vi "Main.vi"(11 "Module Admin":refnum<class "Delacor_lib_QMH_Cloneable Module Admin.lvclass">) -> ()   [LabVIEW 2025, in "Motor.lvlib"]
doc: "This template is based off of the Queued Message Handler design pattern and the Queued Message Handler project template that ships with LabVIEW.\n\nThe main difference is that the queue is private to this module and communication between modules is performed via Broadcast and Request events.\n\nRequest events are wrapped in public API methods and are handled in the Event Handling Loop (EHL) of this VI. Any module can register for Broadcast events sent by this module. The EHL generates messages based on user interface actions.\n\nThe Message Handling Loop (MHL) processes messages generated by the EHL, or by other messages. The messages are string values, so new messages can be added easily to the Message Cases case structure in the MHL. Each message cluster can also provide an optional value for Message Data, which is a variant that can be converted to whatever message-specific data is required.\n_____\nBased on DQMH Dev Tools: Project Template 7.1.2.1547."
uses:
  Motor.lvlib
  <vilib>/Delacor/Delacor QMH/Libraries/Message Queue_class/Delacor_lib_QMH_Message Queue.lvclass
  Module Data--cluster.ctl
  <vilib>/Utility/miscctls.llb/LVPointTypeDef.ctl
  <vilib>/Delacor/Delacor QMH/Libraries/Message Queue_class/Delacor_lib_QMH_Enqueue Message (Single).vi
  Stop Argument--cluster.ctl
  <vilib>/Delacor/Delacor QMH/Libraries/Cloneable Module Admin_class/Delacor_lib_QMH_Cloneable Module Admin.lvclass
  close (Reply Payload)--cluster.ctl
  close Argument--cluster.ctl
  Classes/Stepper/Stepper.lvclass
  init (Reply Payload)--cluster.ctl
  init Argument--cluster.ctl
  clear error (Reply Payload)--cluster.ctl
  clear error Argument--cluster.ctl
  read config (Reply Payload)--cluster.ctl
  read config Argument--cluster.ctl
  read position (Reply Payload)--cluster.ctl
  read position Argument--cluster.ctl
  go to position (Reply Payload)--cluster.ctl
  go to position Argument--cluster.ctl
  jog motor (Reply Payload)--cluster.ctl
  jog motor Argument--cluster.ctl
  select child (Reply Payload)--cluster.ctl
  Classes/Stepper/Motor Selection.ctl
  select child Argument--cluster.ctl
  Classes/CL57RS/CL57RS.lvclass
  C:/Users/Tyson.Grover/Desktop/Repositories/torque-test-station/Libraries/Motor/Classes/Stepper/Stepper.lvclass
  C:/Users/Tyson.Grover/Desktop/Repositories/torque-test-station/Libraries/Motor/Classes/CL57RS/CL57RS.lvclass
panel:
  out "error out":errorcluster
  out "Status":string
  in  "Simulate EHL Error":bool
  in  "Simulate MHL Error":bool
  # "Other processes communicate with this Module via its Public API (wrappers for its Request Events).\n\nThis Module communicates with other processes via its Broadcast Events.\nAny process that wants to receive these messages can register for this module's Broadcast events."
  # "This template is for the DQMH framework. See the block diagram for more information on how to use this template."
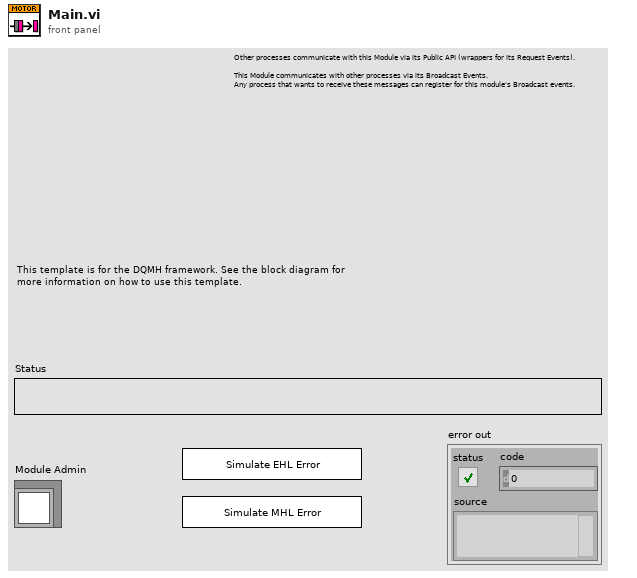
[diagram p1: front panel]
types:
  T1 = typedef "Motor.lvlib/Request Events--cluster.ctl" = cluster{"Stop Module":refnum<user-event>, "Show Panel":refnum<user-event>, "Hide Panel":refnum<user-event>, "Show Diagram":refnum<user-event>, "Get Module Execution Status":refnum<user-event>, "close":refnum<user-event>, "init":refnum<user-event>, "clear error":refnum<user-event>, "read config":refnum<user-event>, "read position":refnum<user-event>, "go to position":refnum<user-event>, "jog motor":refnum<user-event>, "select child":refnum<user-event>}
  T2 = typedef "Motor.lvlib/Module Data--cluster.ctl" = cluster{"Status":string, "Motor Object":refnum<class "Stepper.lvclass">}
  T3 = enum32{"invalid lock state", "Not Locked", "Locked (No Password)", "Password-protected"}
  T4 = typedef "Motor.lvlib/Stop Argument--cluster.ctl" = cluster{"Module ID":i32, "Origin":string, "Exit via Stop Module Req?":bool, "Wait for Module to stop?":bool}
  T5 = typedef "Motor.lvlib/close Argument--cluster.ctl" = cluster{"Module ID":i32, "Wait Notifier":refnum<notifier>, "wait for reply":bool}
  T6 = typedef "Motor.lvlib/init Argument--cluster.ctl" = cluster{"Module ID":i32, "Wait Notifier":refnum<notifier>, "wait for reply":bool}
  T7 = typedef "Motor.lvlib/clear error Argument--cluster.ctl" = cluster{"Module ID":i32, "Wait Notifier":refnum<notifier>, "wait for reply":bool}
  T8 = typedef "Motor.lvlib/read config Argument--cluster.ctl" = cluster{"Module ID":i32, "json file path":path, "Wait Notifier":refnum<notifier>, "wait for reply":bool}
  T9 = typedef "Motor.lvlib/read position Argument--cluster.ctl" = cluster{"Module ID":i32, "Wait Notifier":refnum<notifier>, "wait for reply":bool}
  T10 = typedef "Motor.lvlib/go to position Argument--cluster.ctl" = cluster{"Module ID":i32, "Position":dbl, "Velocity [rpm]":i32, "Pause Time [ms]":i32, "Wait Notifier":refnum<notifier>, "wait for reply":bool}
  T11 = typedef "Motor.lvlib/jog motor Argument--cluster.ctl" = cluster{"Module ID":i32, "CCW? (T)":bool, "Speed [rpm]":dbl, "Wait Notifier":refnum<notifier>, "wait for reply":bool}
  T12 = typedef "Motor.lvlib/select child Argument--cluster.ctl" = cluster{"Module ID":i32, "Enum":T13, "Wait Notifier":refnum<notifier>, "wait for reply":bool}
  T13 = typedef "Motor Selection.ctl" = enum16{"Stepper", "CL57RS"}
  T14 = typedef "LVPointTypeDef.ctl" = cluster{"Horizontal":i16, "Vertical":i16}
  T15 = enum32{"Invalid", "Standard", "Closed", "Hidden", "Minimized", "Maximized"}
  T16 = typedef "Motor.lvlib/close (Reply Payload)--cluster.ctl" = cluster{"Module ID":i32, "error":errorcluster}
  T17 = typedef "Motor.lvlib/init (Reply Payload)--cluster.ctl" = cluster{"Module ID":i32, "error":errorcluster}
  T18 = typedef "Motor.lvlib/clear error (Reply Payload)--cluster.ctl" = cluster{"Module ID":i32, "error":errorcluster}
  T19 = typedef "Motor.lvlib/read config (Reply Payload)--cluster.ctl" = cluster{"Module ID":i32, "error":errorcluster}
  T20 = typedef "Motor.lvlib/read position (Reply Payload)--cluster.ctl" = cluster{"Module ID":i32, "Position":dbl, "error":errorcluster}
  T21 = typedef "Motor.lvlib/go to position (Reply Payload)--cluster.ctl" = cluster{"Module ID":i32, "Position":dbl, "error":errorcluster}
  T22 = typedef "Motor.lvlib/jog motor (Reply Payload)--cluster.ctl" = cluster{"Module ID":i32, "Position":dbl, "error":errorcluster}
  T23 = typedef "Motor.lvlib/select child (Reply Payload)--cluster.ctl" = cluster{"Module ID":i32, "error":errorcluster}
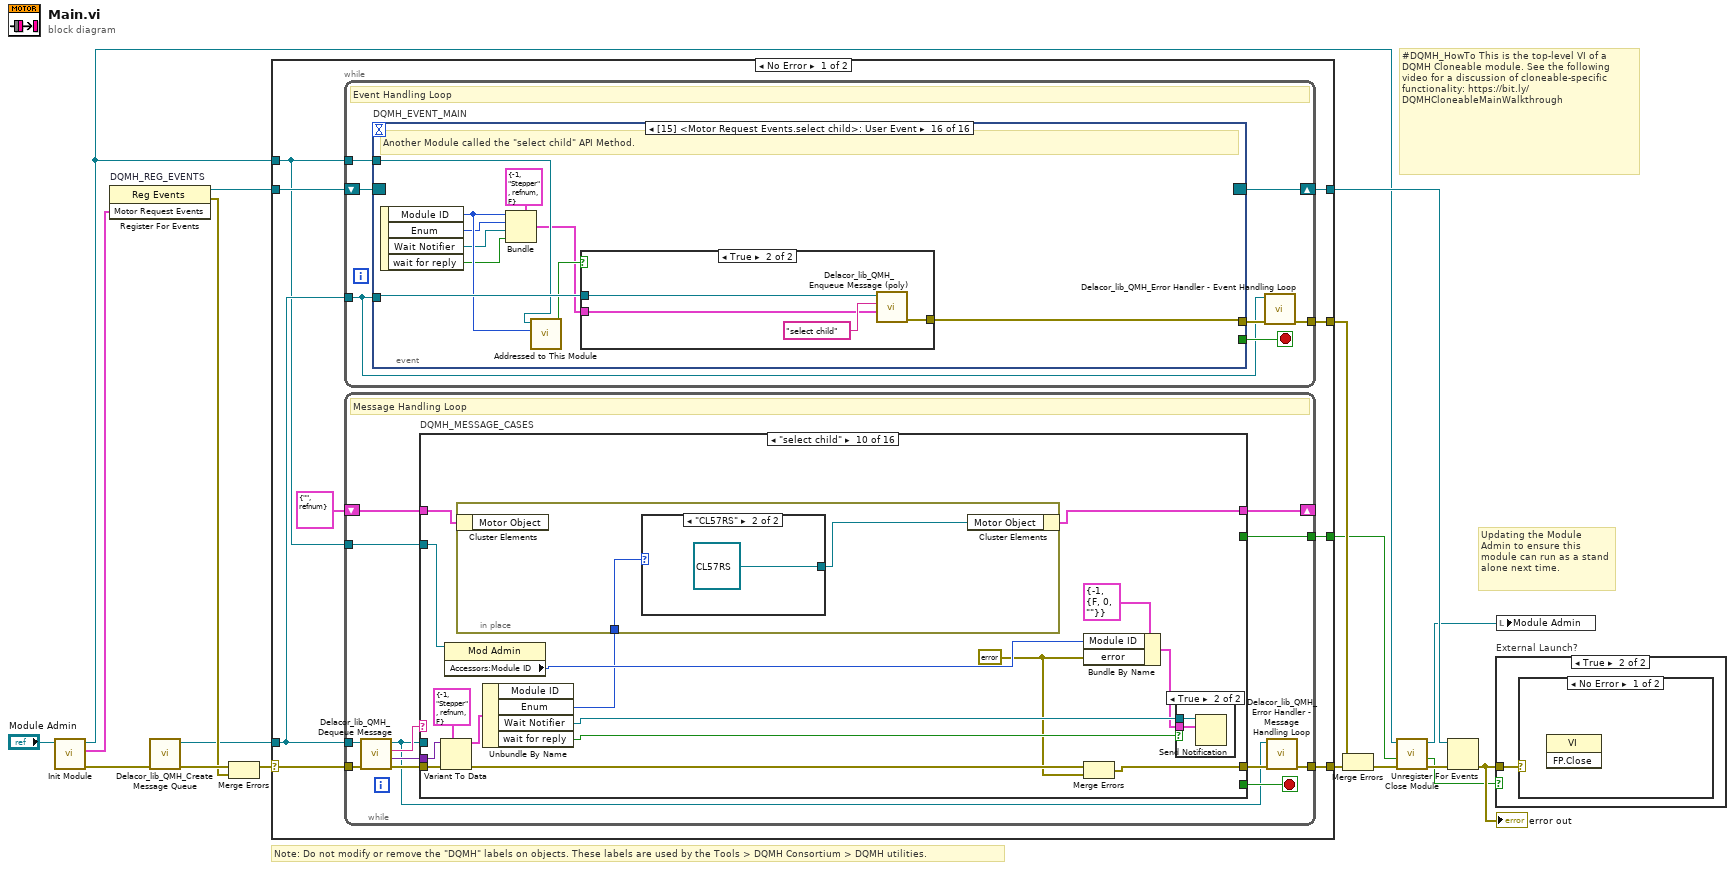
[diagram p0: block diagram]
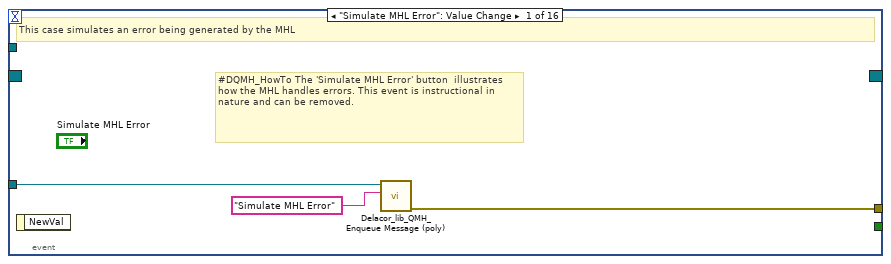
[diagram p2: hidden frame]
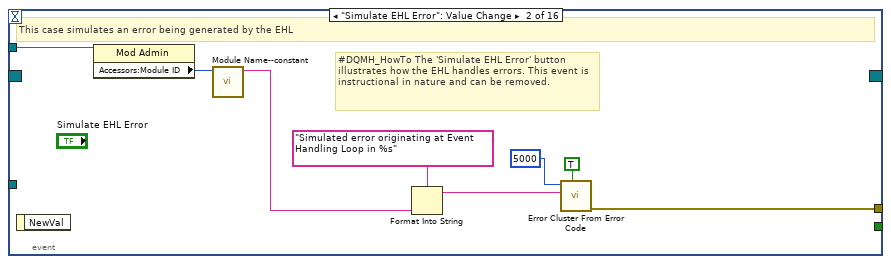
[diagram p3: hidden frame]
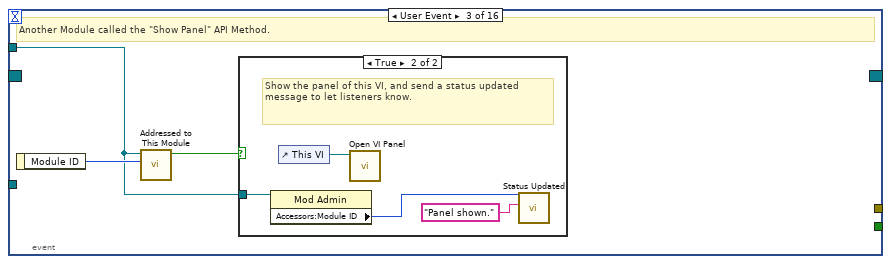
[diagram p4: hidden frame]
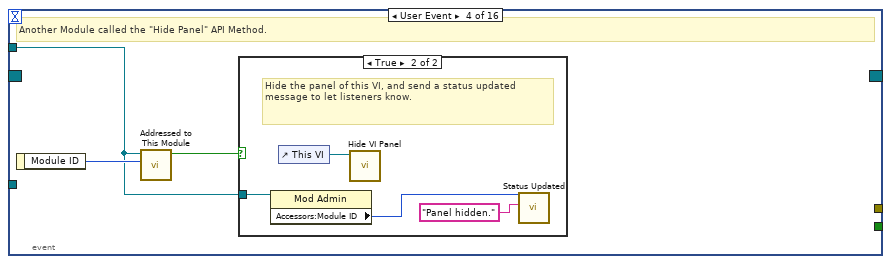
[diagram p6: hidden frame]
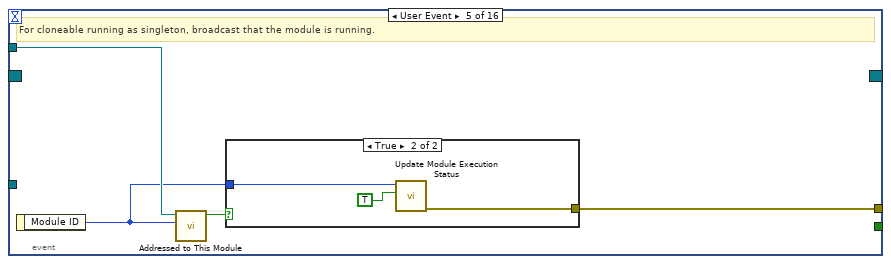
[diagram p8: hidden frame]
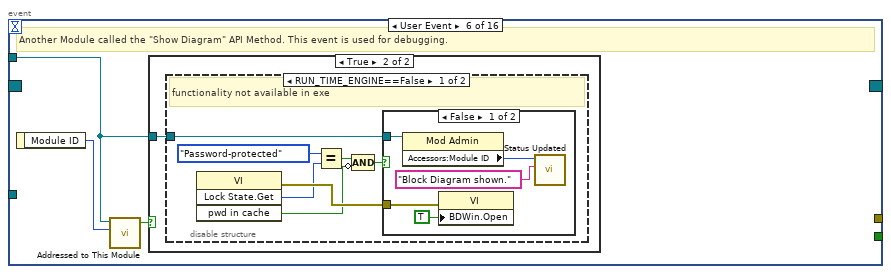
[diagram p10: hidden frame]
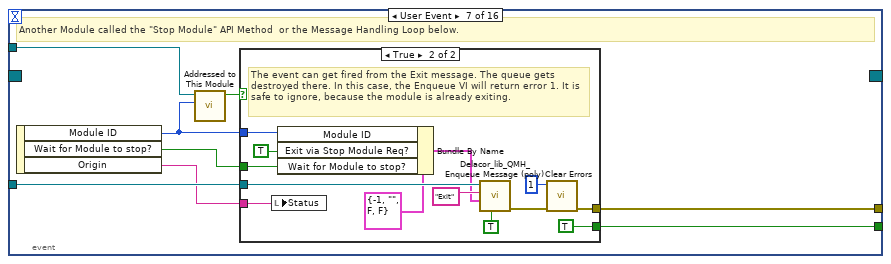
[diagram p14: hidden frame]
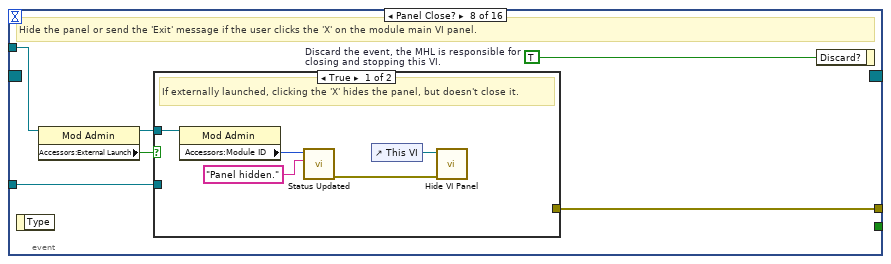
[diagram p16: hidden frame]
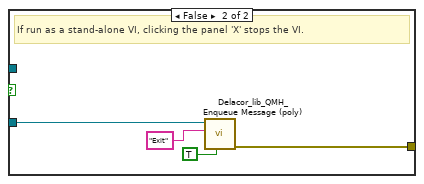
[diagram p17: hidden frame]
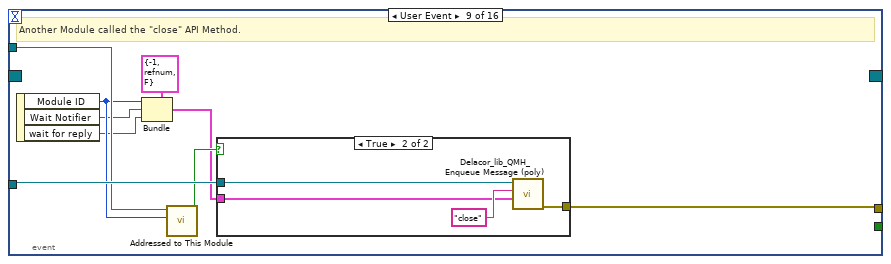
[diagram p18: hidden frame]
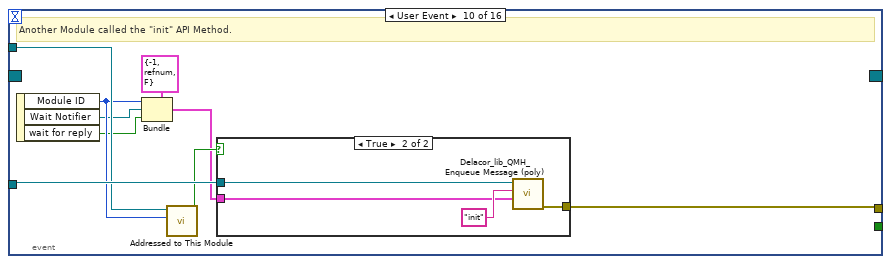
[diagram p20: hidden frame]
diagram:
  # "#DQMH_HowTo This is the top-level VI of a DQMH Cloneable module. See the following video for a discussion of cloneable-specific functionality: https://bit.ly/DQMHCloneableMainWalkthrough"
  # "Note: Do not modify or remove the \"DQMH\" labels on objects. These labels are used by the Tools > DQMH Consortium > DQMH utilities."
  # "Updating the Module Admin to ensure this module can run as a stand alone next time."
  n1 = call "Init Module.vi"("Cloneable Module Admin in"="Module Admin") -> ("error out"=w15:errorcluster, "Motor Request Events"=w7:T1, "Cloneable Module Admin out"=w4:refnum<class "Delacor_lib_QMH_Cloneable Module Admin.lvclass">)  [unwired: 8 in]
  n2 = register-events "DQMH_REG_EVENTS"(w7) -> (reference out=w8:refnum<event-registration>, error out=w10:errorcluster)  [unwired: 2 in]
  n3 = call <vilib>:"Delacor_lib_QMH_Create Message Queue.vi"("error in"=w15) -> ("error out"=w12:errorcluster, "Message Queue"=w6:refnum<class "Delacor_lib_QMH_Message Queue.lvclass">)  [unwired: 9 in]
  n4 = Merge Errors(w12, w10) -> (w11:errorcluster)
  n5 = case shown="No Error" w11 {
    selector: w11 -> [w25 w524]
    tunnel: [w27 w523] -> w16
    tunnel: [w24 w522] -> w9
    tunnel: w8 -> [w22 w522]
    tunnel: w6 -> [w21 w515]
    tunnel: [w26 _] -> w17
    tunnel: w4 -> [w20 w518]
    tunnel: [w19 _] -> w2
    frame No Error {
      n6 = while {
        tunnel: w21 -> [w28]
        shift-right: [w31] -> w24
        shift-left: w22 -> [w32]
        tunnel: [w33] -> w26
        tunnel: w20 -> [w29]
        stop <- w30 stop-if-true
        # "Event Handling Loop"
        n7 = event "DQMH_EVENT_MAIN" shown="[15] <Motor Request Events.select child>: User Event" {
          selector: w32 -> [_ _ _ _ _ _ _ _ _ _ _ _ _ _ _ _]
          dyn-events: [_ _ _ _ _ _ _ _ _ _ _ _ _ _ _ _] -> w31
          timeout: _ -> [_ _ _ _ _ _ _ _ _ _ _ _ _ _ _ _]
          tunnel: [_ _ _ _ _ _ w86 _ _ _ _ _ _ _ _ _] -> w30
          tunnel: w28 -> [w36 _ _ _ _ _ w89 w106 w127 w140 w153 w167 w180 w196 w211 w225]
          tunnel: [w37 w45 _ _ w63 _ w90 w109 w119 w132 w145 w158 w172 w185 w201 w216] -> w34
          tunnel: w29 -> [_ w44 w46 w53 w61 w67 w88 w107 w125 w138 w151 w165 w178 w194 w209 w223]
          event "Simulate MHL Error": Value Change {
            # "#DQMH_HowTo The 'Simulate MHL Error' button  illustrates how the MHL handles errors. This event is instructional in nature and can be removed."
            # "This case simulates an error being generated by the MHL"
            n8 = event-data() -> ()  [unwired: 1 in, 1 out]
            n9 = call-poly <vilib>:"Delacor_lib_QMH_Enqueue Message (poly).vi"("Message"="Simulate MHL Error", "Message Queue in"=w36) -> ("error out"=w37:errorcluster)  [unwired: 8 in, 1 out]
          }
          event "Simulate EHL Error": Value Change {
            # "#DQMH_HowTo The 'Simulate EHL Error' button  illustrates how the EHL handles errors. This event is instructional in nature and can be removed."
            # "This case simulates an error being generated by the EHL"
            n10 = event-data() -> ()  [unwired: 1 in, 1 out]
            n11 = property on="Property Node" class="Mod Admin"(reference=w44) -> ("Accessors:Module ID"=w43:i32)  [unwired: 1 in, 2 out]
            n12 = call "Module Name--constant.vi"("Module ID"=w43) -> ("Module Name"=w38:string)  [unwired: 10 in]
            n13 = Format Into String(format string="Simulated error originating at Event Handling Loop in %s", w38) -> (resulting string=w41:string)  [unwired: 2 in, 1 out]
            n14 = call <vilib>:"Error Cluster From Error Code.vi"("show call chain? (False)"=TRUE, "error message (\"\")"=w41, "error code (0)"=5000) -> ("error out"=w45:errorcluster)  [unwired: 6 in]
          }
          event User Event {
            # "Another Module called the \"Show Panel\" API Method."
            n15 = event-data() -> ("Module ID"=w47:i32)  [unwired: 1 in]
            n16 = call "Addressed to This Module.vi"("Module ID from Argument"=w47, "Module Admin"=w46) -> ("Addressed to this instance?"=w48:bool)  [unwired: 8 in, 1 out]
            n17 = case shown="True" w48 {
              tunnel: w46 -> [_ w50]
              frame False {
              }
              frame True {
                # "Show the panel of this VI, and send a status updated message to let listeners know."
                n18 = property on="Property Node" class="Mod Admin"(reference=w50) -> ("Accessors:Module ID"=w49:i32)  [unwired: 1 in, 2 out]
                n19 = control-ref of="This VI"() -> (w52:refnum<vi>)
                n20 = call "Open VI Panel.vi"("VI"=w52) -> ()  [unwired: 10 in, 1 out]
                n21 = call "Status Updated.vi"("Status"="Panel shown." ("format string"), "Module ID"=w49) -> ()  [unwired: 9 in, 1 out]
              }
            }
          }
          event User Event {
            # "Another Module called the \"Hide Panel\" API Method."
            n22 = event-data() -> ("Module ID"=w54:i32)  [unwired: 1 in]
            n23 = call "Addressed to This Module.vi"("Module ID from Argument"=w54, "Module Admin"=w53) -> ("Addressed to this instance?"=w55:bool)  [unwired: 8 in, 1 out]
            n24 = case shown="True" w55 {
              tunnel: w53 -> [_ w57]
              frame False {
              }
              frame True {
                # "Hide the panel of this VI, and send a status updated message to let listeners know."
                n25 = property on="Property Node" class="Mod Admin"(reference=w57) -> ("Accessors:Module ID"=w56:i32)  [unwired: 1 in, 2 out]
                n26 = control-ref of="This VI"() -> (w59:refnum<vi>)
                n27 = call "Hide VI Panel.vi"("VI"=w59) -> ()  [unwired: 10 in, 1 out]
                n28 = call "Status Updated.vi"("Status"="Panel hidden." ("format string"), "Module ID"=w56) -> ()  [unwired: 9 in, 1 out]
              }
            }
          }
          event User Event {
            # "For cloneable running as singleton, broadcast that the module is running."
            n29 = event-data() -> ("Module ID"=w60:i32)  [unwired: 1 in]
            n30 = call "Addressed to This Module.vi"("Module ID from Argument"=w60, "Module Admin"=w61) -> ("Addressed to this instance?"=w62:bool)  [unwired: 8 in, 1 out]
            n31 = case shown="True" w62 {
              tunnel: [_ w66] -> w63
              tunnel: w60 -> [_ w65]
              frame False {
              }
              frame True {
                n32 = call "Update Module Execution Status.vi"("Running?"=TRUE, "Module ID"=w65) -> ("error out"=w66:errorcluster)  [unwired: 9 in]
              }
            }
          }
          event User Event {
            # "Another Module called the \"Show Diagram\" API Method. This event is used for debugging."
            n33 = event-data() -> ("Module ID"=w68:i32)  [unwired: 1 in]
            n34 = call "Addressed to This Module.vi"("Module ID from Argument"=w68, "Module Admin"=w67) -> ("Addressed to this instance?"=w69:bool)  [unwired: 8 in, 1 out]
            n35 = case shown="True" w69 {
              tunnel: w67 -> [_ w70]
              frame False {
              }
              frame True {
                n36 = disable-structure shown="RUN_TIME_ENGINE==False" {
                  disable-tunnel: w70 -> [w71 _]
                  frame condition #0 (active) {
                    # "functionality not available in exe"
                    n37 = invoke on="Invoke Node" class="VI" method="Lock State.Get"() -> (error out=w77:errorcluster, "Get Lock State"=w76:T3, "pwd in cache"=w73:bool)  [unwired: 4 in, 1 out]
                    n38 = Equal?(x=T3."Password-protected", y=w76) -> (x = y?=w74:bool)
                    n39 = Compound Arithmetic op=AND(w74, invert w73) -> (w72:bool)
                    n40 = case shown="False" w72 {
                      tunnel: w77 -> [w82 _]
                      tunnel: w71 -> [w79 _]
                      frame False {
                        n41 = property on="Property Node" class="Mod Admin"(reference=w79) -> ("Accessors:Module ID"=w78:i32)  [unwired: 1 in, 2 out]
                        n42 = property on="Property Node" class="VI"(error in=w82, "BDWin.Open"=TRUE ("Block Diagram Window:Open")) -> ()  [unwired: 1 in, 2 out]
                        n43 = call "Status Updated.vi"("Status"="Block Diagram shown." ("format string"), "Module ID"=w78) -> ()  [unwired: 9 in, 1 out]
                      }
                      frame True {
                        # "Password-protected VI, and the password is not in the cache. Do not show the diagram."
                      }
                    }
                  }
                  frame condition #1 {
                  }
                }
              }
            }
          }
          event User Event {
            # "Another Module called the \"Stop Module\" API Method  or the Message Handling Loop below."
            n44 = event-data() -> ("Module ID"=w84:i32, "Wait for Module to stop?"=w85:bool, "Origin"=w83:string)  [unwired: 1 in]
            n45 = call "Addressed to This Module.vi"("Module ID from Argument"=w84, "Module Admin"=w88) -> ("Addressed to this instance?"=w87:bool)  [unwired: 8 in, 1 out]
            n46 = case shown="True" w87 {
              tunnel: [_ w102] -> w90
              tunnel: w89 -> [_ w98]
              tunnel: [_ TRUE] -> w86
              tunnel: w85 -> [_ w93]
              tunnel: w84 -> [_ w95]
              tunnel: w83 -> [_ w91]
              frame False {
              }
              frame True {
                # "The event can get fired from the Exit message. The queue gets destroyed there. In this case, the Enqueue VI will return error 1. It is safe to ignore, because the module is already exiting."
                n47 = local write "Status"(w91) -> ()
                n48 = Bundle By Name(cluster=T4 {"Module ID"=-1, "Origin"="", "Exit via Stop Module Req?"=FALSE, "Wait for Module to stop?"=FALSE} ("Stop Argument"), "Module ID"=w95, "Exit via Stop Module Req?"=TRUE, "Wait for Module to stop?"=w93) -> (w92:T4)
                n49 = call-poly <vilib>:"Delacor_lib_QMH_Enqueue Message (poly).vi"("Priority Message? (F)"=TRUE, "Message Data"=w92, "Message"="Exit", "Message Queue in"=w98) -> ("error out"=w103:errorcluster)  [unwired: 6 in, 1 out]
                n50 = call <vilib>:"Clear Errors.vi"("error in (no error)"=w103, "specific error code to clear (0: all)"=1) -> ("error out"=w102:errorcluster)  [unwired: 4 in, 1 out]
              }
            }
          }
          event Panel Close? {
            w108 = TRUE  # Discard the event, the MHL is responsible for closing and stopping this VI.
            # "Hide the panel or send the 'Exit' message if the user clicks the 'X' on the module main VI panel."
            n51 = event-data() -> ()  [unwired: 1 in, 1 out]
            n52 = property on="Property Node" class="Mod Admin"(reference=w107) -> (reference out=w104:refnum<class "Delacor_lib_QMH_Cloneable Module Admin.lvclass">, "Accessors:External Launch"=w105:bool)  [unwired: 1 in, 1 out]
            n53 = case shown="True" w105 {
              tunnel: w106 -> [_ w117]
              tunnel: [_ w118] -> w109
              tunnel: w104 -> [w112 _]
              frame True {
                # "If externally launched, clicking the 'X' hides the panel, but doesn't close it."
                n54 = property on="Property Node" class="Mod Admin"(reference=w112) -> ("Accessors:Module ID"=w111:i32)  [unwired: 1 in, 2 out]
                n55 = call "Status Updated.vi"("Status"="Panel hidden." ("format string"), "Module ID"=w111) -> ("error out"=w110:errorcluster)  [unwired: 9 in]
                n56 = control-ref of="This VI"() -> (w114:refnum<vi>)
                n57 = call "Hide VI Panel.vi"("error in"=w110, "VI"=w114) -> ()  [unwired: 9 in, 1 out]
              }
              frame False {
                # "If run as a stand-alone VI, clicking the panel 'X' stops the VI."
                n58 = call-poly <vilib>:"Delacor_lib_QMH_Enqueue Message (poly).vi"("Priority Message? (F)"=TRUE, "Message"="Exit", "Message Queue in"=w117) -> ("error out"=w118:errorcluster)  [unwired: 7 in, 1 out]
              }
            }
            n59 = event-data ("Event Filter Node")("Discard?"=w108) -> ()  [unwired: 1 in, 1 out]
          }
          event User Event {
            # "Another Module called the \"close\" API Method."
            n60 = event-data() -> ("Module ID"=w122:i32, "Wait Notifier"=w121:refnum<notifier>, "wait for reply"=w120:bool)  [unwired: 1 in]
            n61 = Bundle(cluster=T5 {"Module ID"=-1, "Wait Notifier"=refnum, "wait for reply"=FALSE} ("close Argument"), "Module ID"=w122, "Wait Notifier"=w121, "wait for reply"=w120) -> (w123:T5)
            n62 = call "Addressed to This Module.vi"("Module ID from Argument"=w122, "Module Admin"=w125) -> ("Addressed to this instance?"=w126:bool)  [unwired: 8 in, 1 out]
            n63 = case shown="True" w126 {
              tunnel: w127 -> [_ w131]
              tunnel: w123 -> [_ w129]
              tunnel: [_ w128] -> w119
              frame False {
              }
              frame True {
                n64 = call-poly <vilib>:"Delacor_lib_QMH_Enqueue Message (poly).vi"("Message Data"=w129, "Message"="close", "Message Queue in"=w131) -> ("error out"=w128:errorcluster)  [unwired: 7 in, 1 out]
              }
            }
          }
          event User Event {
            # "Another Module called the \"init\" API Method."
            n65 = event-data() -> ("Module ID"=w135:i32, "Wait Notifier"=w134:refnum<notifier>, "wait for reply"=w133:bool)  [unwired: 1 in]
            n66 = Bundle(cluster=T6 {"Module ID"=-1, "Wait Notifier"=refnum, "wait for reply"=FALSE} ("init Argument"), "Module ID"=w135, "Wait Notifier"=w134, "wait for reply"=w133) -> (w136:T6)
            n67 = call "Addressed to This Module.vi"("Module ID from Argument"=w135, "Module Admin"=w138) -> ("Addressed to this instance?"=w139:bool)  [unwired: 8 in, 1 out]
            n68 = case shown="True" w139 {
              tunnel: w140 -> [_ w144]
              tunnel: w136 -> [_ w142]
              tunnel: [_ w141] -> w132
              frame False {
              }
              frame True {
                n69 = call-poly <vilib>:"Delacor_lib_QMH_Enqueue Message (poly).vi"("Message Data"=w142, "Message"="init", "Message Queue in"=w144) -> ("error out"=w141:errorcluster)  [unwired: 7 in, 1 out]
              }
            }
          }
          event User Event {
            # "Another Module called the \"clear error\" API Method."
            n70 = event-data() -> ("Module ID"=w148:i32, "Wait Notifier"=w147:refnum<notifier>, "wait for reply"=w146:bool)  [unwired: 1 in]
            n71 = Bundle(cluster=T7 {"Module ID"=-1, "Wait Notifier"=refnum, "wait for reply"=FALSE} ("clear error Argument"), "Module ID"=w148, "Wait Notifier"=w147, "wait for reply"=w146) -> (w149:T7)
            n72 = call "Addressed to This Module.vi"("Module ID from Argument"=w148, "Module Admin"=w151) -> ("Addressed to this instance?"=w152:bool)  [unwired: 8 in, 1 out]
            n73 = case shown="True" w152 {
              tunnel: w153 -> [_ w157]
              tunnel: w149 -> [_ w155]
              tunnel: [_ w154] -> w145
              frame False {
              }
              frame True {
                n74 = call-poly <vilib>:"Delacor_lib_QMH_Enqueue Message (poly).vi"("Message Data"=w155, "Message"="clear error", "Message Queue in"=w157) -> ("error out"=w154:errorcluster)  [unwired: 7 in, 1 out]
              }
            }
          }
          event User Event {
            # "Another Module called the \"read config\" API Method."
            n75 = event-data() -> ("Module ID"=w162:i32, "json file path"=w161:path, "Wait Notifier"=w160:refnum<notifier>, "wait for reply"=w159:bool)  [unwired: 1 in]
            n76 = Bundle(cluster=T8 {"Module ID"=-1, "json file path"=path "", "Wait Notifier"=refnum, "wait for reply"=FALSE} ("read config Argument"), "Module ID"=w162, "json file path"=w161, "Wait Notifier"=w160, "wait for reply"=w159) -> (w163:T8)
            n77 = call "Addressed to This Module.vi"("Module ID from Argument"=w162, "Module Admin"=w165) -> ("Addressed to this instance?"=w166:bool)  [unwired: 8 in, 1 out]
            n78 = case shown="True" w166 {
              tunnel: w167 -> [_ w171]
              tunnel: w163 -> [_ w169]
              tunnel: [_ w168] -> w158
              frame False {
              }
              frame True {
                n79 = call-poly <vilib>:"Delacor_lib_QMH_Enqueue Message (poly).vi"("Message Data"=w169, "Message"="read config", "Message Queue in"=w171) -> ("error out"=w168:errorcluster)  [unwired: 7 in, 1 out]
              }
            }
          }
          event User Event {
            # "Another Module called the \"read position\" API Method."
            n80 = event-data() -> ("Module ID"=w175:i32, "Wait Notifier"=w174:refnum<notifier>, "wait for reply"=w173:bool)  [unwired: 1 in]
            n81 = Bundle(cluster=T9 {"Module ID"=-1, "Wait Notifier"=refnum, "wait for reply"=FALSE} ("read position Argument"), "Module ID"=w175, "Wait Notifier"=w174, "wait for reply"=w173) -> (w176:T9)
            n82 = call "Addressed to This Module.vi"("Module ID from Argument"=w175, "Module Admin"=w178) -> ("Addressed to this instance?"=w179:bool)  [unwired: 8 in, 1 out]
            n83 = case shown="True" w179 {
              tunnel: w180 -> [_ w184]
              tunnel: w176 -> [_ w182]
              tunnel: [_ w181] -> w172
              frame False {
              }
              frame True {
                n84 = call-poly <vilib>:"Delacor_lib_QMH_Enqueue Message (poly).vi"("Message Data"=w182, "Message"="read position", "Message Queue in"=w184) -> ("error out"=w181:errorcluster)  [unwired: 7 in, 1 out]
              }
            }
          }
          event User Event {
            # "Another Module called the \"go to position\" API Method."
            n85 = event-data() -> ("Module ID"=w191:i32, "Position"=w190:dbl, "Velocity [rpm]"=w189:i32, "Pause Time [ms]"=w188:i32, "Wait Notifier"=w187:refnum<notifier>, "wait for reply"=w186:bool)  [unwired: 1 in]
            n86 = Bundle(cluster=T10 {"Module ID"=-1, "Position"=0.0, "Velocity [rpm]"=5, "Pause Time [ms]"=50, "Wait Notifier"=refnum, "wait for reply"=FALSE} ("jog Argument"), "Module ID"=w191, "Position"=w190, "Velocity [rpm]"=w189, "Pause Time [ms]"=w188, "Wait Notifier"=w187, "wait for reply"=w186) -> (w192:T10)
            n87 = call "Addressed to This Module.vi"("Module ID from Argument"=w191, "Module Admin"=w194) -> ("Addressed to this instance?"=w195:bool)  [unwired: 8 in, 1 out]
            n88 = case shown="True" w195 {
              tunnel: w196 -> [_ w200]
              tunnel: w192 -> [_ w198]
              tunnel: [_ w197] -> w185
              frame False {
              }
              frame True {
                n89 = call-poly <vilib>:"Delacor_lib_QMH_Enqueue Message (poly).vi"("Message Data"=w198, "Message"="jog", "Message Queue in"=w200) -> ("error out"=w197:errorcluster)  [unwired: 7 in, 1 out]
              }
            }
          }
          event User Event {
            # "Another Module called the \"jog motor\" API Method."
            n90 = event-data() -> ("Module ID"=w206:i32, "CCW? (T)"=w205:bool, "Speed [rpm]"=w204:dbl, "Wait Notifier"=w203:refnum<notifier>, "wait for reply"=w202:bool)  [unwired: 1 in]
            n91 = Bundle(cluster=T11 {"Module ID"=-1, "CCW? (T)"=TRUE, "Speed [rpm]"=0.0, "Wait Notifier"=refnum, "wait for reply"=FALSE} ("jog motor Argument"), "Module ID"=w206, "CCW? (T)"=w205, "Speed [rpm]"=w204, "Wait Notifier"=w203, "wait for reply"=w202) -> (w207:T11)
            n92 = call "Addressed to This Module.vi"("Module ID from Argument"=w206, "Module Admin"=w209) -> ("Addressed to this instance?"=w210:bool)  [unwired: 8 in, 1 out]
            n93 = case shown="True" w210 {
              tunnel: w211 -> [_ w215]
              tunnel: w207 -> [_ w213]
              tunnel: [_ w212] -> w201
              frame False {
              }
              frame True {
                n94 = call-poly <vilib>:"Delacor_lib_QMH_Enqueue Message (poly).vi"("Message Data"=w213, "Message"="jog motor", "Message Queue in"=w215) -> ("error out"=w212:errorcluster)  [unwired: 7 in, 1 out]
              }
            }
          }
          event User Event {
            # "Another Module called the \"select child\" API Method."
            n95 = event-data() -> ("Module ID"=w220:i32, "Enum"=w219:T13, "Wait Notifier"=w218:refnum<notifier>, "wait for reply"=w217:bool)  [unwired: 1 in]
            n96 = Bundle(cluster=T12 {"Module ID"=-1, "Enum"=enum."Stepper", "Wait Notifier"=refnum, "wait for reply"=FALSE} ("select child Argument"), "Module ID"=w220, "Enum"=w219, "Wait Notifier"=w218, "wait for reply"=w217) -> (w221:T12)
            n97 = call "Addressed to This Module.vi"("Module ID from Argument"=w220, "Module Admin"=w223) -> ("Addressed to this instance?"=w224:bool)  [unwired: 8 in, 1 out]
            n98 = case shown="True" w224 {
              tunnel: w225 -> [_ w229]
              tunnel: w221 -> [_ w227]
              tunnel: [_ w226] -> w216
              frame False {
              }
              frame True {
                n99 = call-poly <vilib>:"Delacor_lib_QMH_Enqueue Message (poly).vi"("Message Data"=w227, "Message"="select child", "Message Queue in"=w229) -> ("error out"=w226:errorcluster)  [unwired: 7 in, 1 out]
              }
            }
          }
        }
        n100 = call-dynamic "Delacor_lib_QMH_Error Handler - Event Handling Loop.vi"("error in"=w34, "Message Queue in"=w28) -> ("dup error in"=w33:errorcluster)  [unwired: 8 in, 1 out]
      }
      n101 = while {
        tunnel: w21 -> [w230]
        shift-right: [w237] -> _
        shift-left: T2 {"Status"="", "Motor Object"=refnum} ("Data Cluster") -> [w238]
        tunnel: w25 -> [w241]
        tunnel: [w239] -> w27
        tunnel: w20 -> [w232]
        tunnel: [w231] -> w19
        stop <- w236 stop-if-true
        # "Message Handling Loop"
        n102 = call-dynamic "Delacor_lib_QMH_Dequeue Message.vi"("error in"=w241, "Message Queue in"=w230) -> ("error out"=w240:errorcluster, "Message Data"=w234:variant, "Message"=w235:string, "Message Queue out"=w233:refnum<class "Delacor_lib_QMH_Message Queue.lvclass">)  [unwired: 6 in]
        n103 = case "DQMH_MESSAGE_CASES" shown="\"select child\"" w235 {
          selector: w235 -> [_ _ _ _ _ _ _ _ _ _ _ _ _ _ _ w504]
          tunnel: w233 -> [_ _ _ _ _ _ _ _ _ _ _ _ w459 _ w496 _]
          tunnel: w240 -> [w261 w265 w280 w300 w320 w341 w363 w388 w417 w445 w454 w456 w468 w485 w502 w513]
          tunnel: [w259 w265 w271 w291 w311 w332 w354 w379 w408 w436 w453 w456 w464 w484 w497 w514] -> w242
          tunnel: w238 -> [w252 w264 w268 w288 w308 w329 w351 w376 w405 w433 w452 w455 w463 w482 w495 w511]
          tunnel: [w251 w264 w267 w287 w307 w328 w350 w375 w404 w431 w452 w455 w463 w482 w495 w511] -> w237
          tunnel: [_ _ _ _ _ _ _ _ _ _ _ _ _ _ w494 _] -> w236
          tunnel: w234 -> [_ _ w278 w298 w318 w339 w361 w386 w415 w443 _ _ w462 _ w492 _]
          tunnel: w232 -> [w247 _ w269 w289 w309 w330 w352 w377 w406 w434 _ _ w461 w480 w487 w510]
          tunnel: [_ _ _ _ _ _ _ _ _ _ _ _ _ _ w490 _] -> w231
          frame "Initialize" {
            w244 = "Initial Message" ("Initial Message")
            # "#DQMH_CodeNeeded - Initialize the appearance of the front panel."
            # "#DQMH_CodeNeeded - Initialize your state data here."
            # "Initialize - Any operation that needs to be done before the module can receive messages. Synchronize Caller Events.vi will inform Start Module.vi that the module has launched and is ready to receive messages. Module Did Init.vi will broadcast that the module initialized."
            n104 = call "Synchronize Caller Events.vi"("error in"=w261, "Module Admin"=w247) -> ("error out"=w260:errorcluster, "Module Admin out"=w246:refnum<class "Delacor_lib_QMH_Cloneable Module Admin.lvclass">)  [unwired: 8 in]
            n105 = property on="Property Node" class="Mod Admin"(reference=w246) -> ("Accessors:Module ID"=w243:i32, "Accessors:External Launch"=w248:bool)  [unwired: 1 in, 2 out]
            n106 = call "Module Name--constant.vi"("Module ID"=w243) -> ("Module Name"=w256:string)  [unwired: 10 in]
            n107 = property on="Property Node" class="VI"("Front Panel.Title"=w256) -> (reference out=w258:refnum<vi>, error out=w263:errorcluster)  [unwired: 2 in]
            n108 = Select(t=T15."Hidden" ("State"), s=w248, f=T15."Standard" ("State")) -> (s? t:f=w253:T15)
            n109 = invoke on="Invoke Node" class="VI" method="FP.Open"(reference=w258, error in=w263, "State"=w253) -> (reference out=w257:refnum<vi>, error out=w262:errorcluster)  [unwired: 2 in, 3 out]
            n110 = Bundle By Name(cluster=w252, "Status"=w244) -> (w251:T2)
            n111 = invoke on="Invoke Node" class="VI" method="FP.Center"(reference=w257, error in=w262) -> ()  [unwired: 1 in, 3 out]
            n112 = property on="Pane" class="Pane"("Origin"=T14 {"Horizontal"=0, "Vertical"=0}) -> ()  [unwired: 2 in, 2 out]
            n113 = call "Module Name--constant.vi"("Module ID"=w243) -> ("Module Name"=w249:string)  [unwired: 10 in]
            n114 = call "Module Did Init.vi"("error in"=w260, "Initialized?"=TRUE, "Origin"=w249, "Module ID"=w243) -> ("error out"=w259:errorcluster)  [unwired: 7 in]
            "Status" <- w244
          }
          frame "---Module Specific---" {
            # "Separator -- The following cases handle messages specific to this Module."
          }
          frame "close" {
            n115 = Variant To Data(error in=w280, type=T5 {"Module ID"=-1, "Wait Notifier"=refnum, "wait for reply"=FALSE} ("close Argument"), Variant=w278) -> (data=w276:T5, error out=w279:errorcluster)
            n116 = property class="Mod Admin"(reference=w269) -> ("Accessors:Module ID"=w270:i32)  [unwired: 1 in, 2 out]
            n117 = in-place {
              in-place-border: [w281] -> w266
              n118 = in-place-cluster #1(w268) -> ("Motor Object"=w282:refnum<class "Stepper.lvclass">)
              n119 = call-dynamic "close.vi"("Stepper in"=w282) -> ("error out"=w281:errorcluster, "Stepper out"=w283:refnum<class "Stepper.lvclass">)  [unwired: 9 in]
              n120 = in-place-cluster #1("Motor Object"=w283) -> (w267:T2)
            }
            n121 = Unbundle By Name(w276) -> ("Wait Notifier"=w275:refnum<notifier>, "wait for reply"=w274:bool)  [unwired: 1 out]
            n122 = Bundle By Name(cluster=T16 {"Module ID"=-1, "error"={"status"=FALSE, "code"=0, "source"=""}} ("close (Reply Payload)"), "Module ID"=w270, "error"=w266) -> (w273:T16)
            n123 = Merge Errors(w279, w266) -> (w271:errorcluster)
            n124 = case "DQMH_FIRE_NOTIFIER" shown="True" w274 {
              tunnel: w275 -> [_ w285]
              tunnel: w273 -> [_ w284]
              frame False {
              }
              frame True {
                n125 = Send Notification(notification=w284, notifier=w285) -> ()  [unwired: 1 in, 2 out]
              }
            }
          }
          frame "init" {
            n126 = property class="Mod Admin"(reference=w289) -> ("Accessors:Module ID"=w290:i32)  [unwired: 1 in, 2 out]
            n127 = Variant To Data(error in=w300, type=T6 {"Module ID"=-1, "Wait Notifier"=refnum, "wait for reply"=FALSE} ("init Argument"), Variant=w298) -> (data=w296:T6, error out=w299:errorcluster)
            n128 = in-place {
              in-place-border: [w301] -> w286
              n129 = in-place-cluster #2(w288) -> ("Motor Object"=w303:refnum<class "Stepper.lvclass">)
              n130 = call-dynamic "init.vi"("Stepper in"=w303) -> ("error out"=w301:errorcluster, "Stepper out"=w302:refnum<class "Stepper.lvclass">)  [unwired: 9 in]
              n131 = in-place-cluster #2("Motor Object"=w302) -> (w287:T2)
            }
            n132 = Unbundle By Name(w296) -> ("Wait Notifier"=w295:refnum<notifier>, "wait for reply"=w294:bool)  [unwired: 1 out]
            n133 = Bundle By Name(cluster=T17 {"Module ID"=-1, "error"={"status"=FALSE, "code"=0, "source"=""}} ("init (Reply Payload)"), "Module ID"=w290, "error"=w286) -> (w293:T17)
            n134 = Merge Errors(w299, w286) -> (w291:errorcluster)
            n135 = case "DQMH_FIRE_NOTIFIER" shown="True" w294 {
              tunnel: w295 -> [_ w305]
              tunnel: w293 -> [_ w304]
              frame False {
              }
              frame True {
                n136 = Send Notification(notification=w304, notifier=w305) -> ()  [unwired: 1 in, 2 out]
              }
            }
          }
          frame "clear error" {
            n137 = Variant To Data(error in=w320, type=T7 {"Module ID"=-1, "Wait Notifier"=refnum, "wait for reply"=FALSE} ("clear error Argument"), Variant=w318) -> (data=w316:T7, error out=w319:errorcluster)
            n138 = property class="Mod Admin"(reference=w309) -> ("Accessors:Module ID"=w310:i32)  [unwired: 1 in, 2 out]
            n139 = in-place {
              in-place-border: [w321] -> w306
              n140 = in-place-cluster #3(w308) -> ("Motor Object"=w323:refnum<class "Stepper.lvclass">)
              n141 = call-dynamic "clear motor error.vi"("Stepper in"=w323) -> ("error out"=w321:errorcluster, "Stepper out"=w322:refnum<class "Stepper.lvclass">)  [unwired: 9 in]
              n142 = in-place-cluster #3("Motor Object"=w322) -> (w307:T2)
            }
            n143 = Unbundle By Name(w316) -> ("Wait Notifier"=w315:refnum<notifier>, "wait for reply"=w314:bool)  [unwired: 1 out]
            n144 = Bundle By Name(cluster=T18 {"Module ID"=-1, "error"={"status"=FALSE, "code"=0, "source"=""}} ("clear error (Reply Payload)"), "Module ID"=w310, "error"=w306) -> (w313:T18)
            n145 = Merge Errors(w319, w306) -> (w311:errorcluster)
            n146 = case "DQMH_FIRE_NOTIFIER" shown="True" w314 {
              tunnel: w315 -> [_ w325]
              tunnel: w313 -> [_ w324]
              frame False {
              }
              frame True {
                n147 = Send Notification(notification=w324, notifier=w325) -> ()  [unwired: 1 in, 2 out]
              }
            }
          }
          frame "read config" {
            n148 = Variant To Data(error in=w341, type=T8 {"Module ID"=-1, "json file path"=path "", "Wait Notifier"=refnum, "wait for reply"=FALSE} ("read config Argument"), Variant=w339) -> (data=w337:T8, error out=w340:errorcluster)
            n149 = property class="Mod Admin"(reference=w330) -> ("Accessors:Module ID"=w331:i32)  [unwired: 1 in, 2 out]
            n150 = Unbundle By Name(w337) -> ("json file path"=w326:path, "Wait Notifier"=w336:refnum<notifier>, "wait for reply"=w335:bool)  [unwired: 1 out]
            n151 = in-place {
              in-place-border: [w344] -> w327
              in-place-border: w326 -> [w342]
              n152 = in-place-cluster #4(w329) -> ("Motor Object"=w343:refnum<class "Stepper.lvclass">)
              n153 = call-dynamic "read config.vi"("Config File Path"=w342, "Stepper in"=w343) -> ("error out"=w344:errorcluster, "Stepper out"=w345:refnum<class "Stepper.lvclass">)  [unwired: 8 in]
              n154 = in-place-cluster #4("Motor Object"=w345) -> (w328:T2)
            }
            n155 = Bundle By Name(cluster=T19 {"Module ID"=-1, "error"={"status"=FALSE, "code"=0, "source"=""}} ("read config (Reply Payload)"), "Module ID"=w331, "error"=w327) -> (w334:T19)
            n156 = Merge Errors(w340, w327) -> (w332:errorcluster)
            n157 = case "DQMH_FIRE_NOTIFIER" shown="True" w335 {
              tunnel: w336 -> [_ w347]
              tunnel: w334 -> [_ w346]
              frame False {
              }
              frame True {
                n158 = Send Notification(notification=w346, notifier=w347) -> ()  [unwired: 1 in, 2 out]
              }
            }
          }
          frame "read position" {
            n159 = Variant To Data(error in=w363, type=T9 {"Module ID"=-1, "Wait Notifier"=refnum, "wait for reply"=FALSE} ("read position Argument"), Variant=w361) -> (data=w359:T9, error out=w362:errorcluster)
            n160 = property class="Mod Admin"(reference=w352) -> ("Accessors:Module ID"=w353:i32)  [unwired: 1 in, 2 out]
            n161 = in-place {
              in-place-border: [w365] -> w349
              in-place-border: [w364] -> w348
              n162 = in-place-cluster #5(w351) -> ("Motor Object"=w367:refnum<class "Stepper.lvclass">)
              n163 = call-dynamic "read position.vi"("Stepper in"=w367) -> ("error out"=w364:errorcluster, "Angle"=w365:dbl, "Stepper out"=w366:refnum<class "Stepper.lvclass">)  [unwired: 8 in]
              n164 = in-place-cluster #5("Motor Object"=w366) -> (w350:T2)
            }
            n165 = Unbundle By Name(w359) -> ("Wait Notifier"=w358:refnum<notifier>, "wait for reply"=w357:bool)  [unwired: 1 out]
            n166 = Bundle By Name(cluster=T20 {"Module ID"=-1, "Position"=0.0, "error"={"status"=FALSE, "code"=0, "source"=""}} ("read position (Reply Payload)"), "Module ID"=w353, "Position"=w349, "error"=w348) -> (w356:T20)
            n167 = Merge Errors(w362, w348) -> (w354:errorcluster)
            n168 = case "DQMH_FIRE_NOTIFIER" shown="True" w357 {
              tunnel: w358 -> [_ w369]
              tunnel: w356 -> [_ w368]
              frame False {
              }
              frame True {
                n169 = Send Notification(notification=w368, notifier=w369) -> ()  [unwired: 1 in, 2 out]
              }
            }
          }
          frame "jog" {
            n170 = property class="Mod Admin"(reference=w377) -> ("Accessors:Module ID"=w378:i32)  [unwired: 1 in, 2 out]
            n171 = Variant To Data(error in=w388, type=T10 {"Module ID"=-1, "Position"=0.0, "Velocity [rpm]"=5, "Pause Time [ms]"=50, "Wait Notifier"=refnum, "wait for reply"=FALSE} ("jog Argument"), Variant=w386) -> (data=w384:T10, error out=w387:errorcluster)
            n172 = Unbundle By Name(w384) -> ("Position"=w374:dbl, "Velocity [rpm]"=w373:i32, "Pause Time [ms]"=w372:i32, "Wait Notifier"=w383:refnum<notifier>, "wait for reply"=w382:bool)  [unwired: 1 out]
            n173 = in-place {
              in-place-border: w374 -> [w394]
              in-place-border: w373 -> [w393]
              in-place-border: w372 -> [w392]
              in-place-border: [w391] -> w371
              in-place-border: [w390] -> w370
              n174 = in-place-cluster #6(w376) -> ("Motor Object"=w397:refnum<class "Stepper.lvclass">)
              n175 = call-dynamic "go to angle.vi"("Pause Time [ms]"=w392, "Velocity [rpm]"=w393, "Angle"=w394, "Stepper in"=w397) -> ("error out"=w395:errorcluster, "Stepper out"=w396:refnum<class "Stepper.lvclass">)  [unwired: 6 in]
              n176 = call-dynamic "read position.vi"("error in (no error)"=w395, "Stepper in"=w396) -> ("error out"=w390:errorcluster, "Angle"=w391:dbl, "Stepper out"=w389:refnum<class "Stepper.lvclass">)  [unwired: 7 in]
              n177 = in-place-cluster #6("Motor Object"=w389) -> (w375:T2)
            }
            n178 = Bundle By Name(cluster=T21 {"Module ID"=-1, "Position"=0.0, "error"={"status"=FALSE, "code"=0, "source"=""}} ("jog (Reply Payload)"), "Module ID"=w378, "Position"=w371, "error"=w370) -> (w381:T21)
            n179 = Merge Errors(w387, w370) -> (w379:errorcluster)
            n180 = case "DQMH_FIRE_NOTIFIER" shown="True" w382 {
              tunnel: w383 -> [_ w399]
              tunnel: w381 -> [_ w398]
              frame False {
              }
              frame True {
                n181 = Send Notification(notification=w398, notifier=w399) -> ()  [unwired: 1 in, 2 out]
              }
            }
          }
          frame "jog motor" {
            n182 = Variant To Data(error in=w417, type=T11 {"Module ID"=-1, "CCW? (T)"=TRUE, "Speed [rpm]"=0.0, "Wait Notifier"=refnum, "wait for reply"=FALSE} ("jog motor Argument"), Variant=w415) -> (data=w413:T11, error out=w416:errorcluster)
            n183 = property class="Mod Admin"(reference=w406) -> ("Accessors:Module ID"=w407:i32)  [unwired: 1 in, 2 out]
            n184 = Unbundle By Name(w413) -> ("CCW? (T)"=w403:bool, "Speed [rpm]"=w402:dbl, "Wait Notifier"=w412:refnum<notifier>, "wait for reply"=w411:bool)  [unwired: 1 out]
            n185 = in-place {
              in-place-border: w403 -> [w426]
              in-place-border: w402 -> [w425]
              in-place-border: [w419] -> w401
              in-place-border: [w418] -> w400
              n186 = in-place-cluster #7(w405) -> ("Motor Object"=w427:refnum<class "Stepper.lvclass">)
              n187 = call-dynamic "set speed.vi"("Speed [rpm]"=w425, "Stepper in"=w427) -> ("error out"=w423:errorcluster, "Stepper out"=w424:refnum<class "Stepper.lvclass">)  [unwired: 8 in]
              n188 = call-dynamic "jog motor.vi"("error in (no error)"=w423, "CCW? (T)"=w426, "Stepper in"=w424) -> ("error out"=w421:errorcluster, "Stepper out"=w422:refnum<class "Stepper.lvclass">)  [unwired: 7 in]
              n189 = call-dynamic "read position.vi"("error in (no error)"=w421, "Stepper in"=w422) -> ("error out"=w418:errorcluster, "Angle"=w419:dbl, "Stepper out"=w420:refnum<class "Stepper.lvclass">)  [unwired: 7 in]
              n190 = in-place-cluster #7("Motor Object"=w420) -> (w404:T2)
            }
            n191 = Bundle By Name(cluster=T22 {"Module ID"=-1, "Position"=0.0, "error"={"status"=FALSE, "code"=0, "source"=""}} ("jog motor (Reply Payload)"), "Module ID"=w407, "Position"=w401, "error"=w400) -> (w410:T22)
            n192 = Merge Errors(w416, w400) -> (w408:errorcluster)
            n193 = case "DQMH_FIRE_NOTIFIER" shown="True" w411 {
              tunnel: w412 -> [_ w429]
              tunnel: w410 -> [_ w428]
              frame False {
              }
              frame True {
                n194 = Send Notification(notification=w428, notifier=w429) -> ()  [unwired: 1 in, 2 out]
              }
            }
          }
          frame "select child" {
            w430 = errorcluster {"status"=FALSE, "code"=0, "source"=""} ("error")
            n195 = Variant To Data(error in=w445, type=T12 {"Module ID"=-1, "Enum"=enum."Stepper", "Wait Notifier"=refnum, "wait for reply"=FALSE} ("select child Argument"), Variant=w443) -> (data=w441:T12, error out=w444:errorcluster)
            n196 = property class="Mod Admin"(reference=w434) -> ("Accessors:Module ID"=w435:i32)  [unwired: 1 in, 2 out]
            n197 = Unbundle By Name(w441) -> ("Enum"=w432:T13, "Wait Notifier"=w440:refnum<notifier>, "wait for reply"=w439:bool)  [unwired: 1 out]
            n198 = in-place {
              in-place-border: w432 -> [w447]
              n199 = in-place-cluster #8(w433) -> ()  [unwired: 1 out]
              n200 = case shown="\"CL57RS\"" w447 {
                tunnel: [refnum<class "Stepper.lvclass"> refnum ("Motor.lvlib:Stepper.lvclass") refnum<class "CL57RS.lvclass"> refnum ("Motor.lvlib:CL57RS.lvclass")] -> w446
                frame "Stepper", Default {
                }
                frame "CL57RS" {
                }
              }
              n201 = in-place-cluster #8("Motor Object"=w446) -> (w431:T2)
            }
            n202 = Bundle By Name(cluster=T23 {"Module ID"=-1, "error"={"status"=FALSE, "code"=0, "source"=""}} ("select child (Reply Payload)"), "Module ID"=w435, "error"=w430) -> (w438:T23)
            n203 = Merge Errors(w444, w430) -> (w436:errorcluster)
            n204 = case "DQMH_FIRE_NOTIFIER" shown="True" w439 {
              tunnel: w440 -> [_ w451]
              tunnel: w438 -> [_ w450]
              frame False {
              }
              frame True {
                n205 = Send Notification(notification=w450, notifier=w451) -> ()  [unwired: 1 in, 2 out]
              }
            }
          }
          frame "---Copy This Frame---" {
            # "Duplicate this frame when creating new messages.  Change this comment in the duplicated frame to describe this message."
            n206 = Merge Errors(w454) -> (w453:errorcluster)
          }
          frame "---Exit and Error Handling---" {
            # "Separator - the following cases handle errors and exit messages."
          }
          frame "Error" {
            # "#DQMH_CodeRecommended - If the module is running in standalone mode (External Launch = FALSE), this code will pop up an error dialog and call the 'Exit' message if an error occurs. Add more fine-grained error management here."
            # "Error - Check the error message data and respond accordingly. This message is sent by the \"Error Handler\" VIs at the end of each loop in this application."
            n207 = property on="Property Node" class="Mod Admin"(reference=w461) -> ("Accessors:External Launch"=w460:bool, "Accessors:Module ID"=w458:i32)  [unwired: 1 in, 2 out]
            n208 = Variant To Data(error in=w468, type=errorcluster {"status"=FALSE, "code"=0, "source"=""} ("error constant"), Variant=w462) -> (data=w457:errorcluster, error out=w466:errorcluster)
            n209 = local write "error out"(w457) -> ()
            n210 = call "Error Reported.vi"("Error"=w457, "Module ID"=w458) -> ()  [unwired: 9 in, 1 out]
            n211 = case shown="False" w460 {
              tunnel: [w473 _] -> w465
              tunnel: w459 -> [w471 _]
              tunnel: w457 -> [w472 _]
              frame False {
                n212 = disable-structure shown="Default" {
                  disable-tunnel: w472 -> [w474 _]
                  frame condition #0 (active) {
                    # "If the module is running standalone, then pop up an error dialog and call the \"Exit\" message."
                    n213 = call <vilib>:"Simple Error Handler.vi"("error in (no error)"=w474) -> ()  [unwired: 4 in, 5 out]
                  }
                  frame condition #1 {
                    # "To prevent the Simple Error Handler VI from being loaded (e.g. when deploying to a Real-Time target), add the Conditional Disable Symbol \"DQMH_Disable_SEH\" to your project and set it to TRUE."
                  }
                }
                n214 = call-poly <vilib>:"Delacor_lib_QMH_Enqueue Message (poly).vi"("Priority Message? (F)"=TRUE, "Message"="Exit", "Message Queue in"=w471) -> ("error out"=w473:errorcluster)  [unwired: 7 in, 1 out]
              }
              frame True {
                # "If the module was launched externally, calling the Error Reported broadcast VI is the only action performed by the \"Error\" message. The module's caller can then process the error appropriately."
              }
            }
            n215 = Merge Errors(w466, w465) -> (w464:errorcluster)
          }
          frame "Simulate MHL Error" {
            # "#DQMH_HowTo The 'Simulate MHL Error' button  illustrates how the MHL handles errors. This event is instructional in nature and can be removed."
            # "Simulate an error occurring at the MHL"
            n216 = property on="Property Node" class="Mod Admin"(reference=w480) -> ("Accessors:Module ID"=w481:i32)  [unwired: 1 in, 2 out]
            n217 = call "Module Name--constant.vi"("Module ID"=w481) -> ("Module Name"=w476:string)  [unwired: 10 in]
            n218 = Format Into String(format string="Simulated error originating at Message Handling Loop in %s", w476) -> (resulting string=w477:string)  [unwired: 2 in, 1 out]
            n219 = call <vilib>:"Error Cluster From Error Code.vi"("show call chain? (False)"=TRUE, "error message (\"\")"=w477, "error code (0)"=5001) -> ("error out"=w483:errorcluster)  [unwired: 6 in]
            n220 = Merge Errors(w485, w483) -> (w484:errorcluster)
          }
          frame "Exit" {
            w493 = 91  # 91: not all Exit messages will have an argument
            w494 = TRUE  # Stop the VI
            # "Release the message queue reference"
            # "#DQMH_CodeNeeded - Add any required cleanup code here."
            # "Exit - Exit the application."
            n221 = Variant To Data(error in=w502, type=T4 {"Module ID"=-1, "Origin"="", "Exit via Stop Module Req?"=FALSE, "Wait for Module to stop?"=FALSE} ("Stop Argument"), Variant=w492) -> (data=w489:T4, error out=w498:errorcluster)
            n222 = call <vilib>:"Clear Errors.vi"("error in (no error)"=w498, "specific error code to clear (0: all)"=w493) -> ("error out"=w501:errorcluster)  [unwired: 4 in, 1 out]
            n223 = property on="Property Node" class="Mod Admin"(reference=w487) -> ("Accessors:Module ID"=w486:i32)  [unwired: 1 in, 2 out]
            n224 = control-ref of="This VI"() -> (w488:refnum<vi>)
            n225 = call-dynamic "Delacor_lib_QMH_Release Message Queue.vi"("error in"=w501, "Message Queue"=w496) -> ("error out"=w500:errorcluster)  [unwired: 9 in]
            n226 = call "Handle Exit.vi"("Stop Argument"=w489, "Module Admin in"=w487, "VI reference"=w488) -> ("error out"=w499:errorcluster, "Wait for Stop?"=w490:bool)  [unwired: 7 in]
            n227 = Merge Errors(w500, w499) -> (w497:errorcluster)
            n228 = call "Error Reported.vi"("Error"=w497, "Module ID"=w486) -> ()  [unwired: 9 in, 1 out]
          }
          frame Default {
            # "'Default' case only runs if there is a message that isn't defined in any of the other cases.  Output a programming error."
            n229 = property on="Property Node" class="Mod Admin"(reference=w510) -> ("Accessors:Module ID"=w509:i32)  [unwired: 1 in, 2 out]
            n230 = call "Module Name--constant.vi"("Module ID"=w509) -> ("Module Name"=w503:string)  [unwired: 10 in]
            n231 = Format Into String(format string="The invalid message string \"%s\" was received in the Message Handling Loop for module \"%s\".", w504, w503) -> (resulting string=w506:string)  [unwired: 2 in, 1 out]
            n232 = call <vilib>:"Error Cluster From Error Code.vi"("show call chain? (False)"=TRUE, "error message (\"\")"=w506, "error code (0)"=1) -> ("error out"=w512:errorcluster)  [unwired: 6 in]
            n233 = Merge Errors(w513, w512) -> (w514:errorcluster)
          }
        }
        n234 = call-dynamic "Delacor_lib_QMH_Error Handler - Message Handling Loop.vi"("error in"=w242, "Message Queue in"=w233) -> ("dup error in"=w239:errorcluster)  [unwired: 8 in, 1 out]
      }
    }
    frame Error {
      n235 = call "Synchronize Caller Events.vi"("Module Admin"=w518) -> ("Module Admin out"=w517:refnum<class "Delacor_lib_QMH_Cloneable Module Admin.lvclass">)  [unwired: 9 in, 1 out]
      n236 = property on="Property Node" class="Mod Admin"(reference=w517) -> ("Accessors:Module ID"=w516:i32)  [unwired: 1 in, 2 out]
      n237 = call-dynamic "Delacor_lib_QMH_Release Message Queue.vi"("error in"=w524, "Message Queue"=w515) -> ("error out"=w523:errorcluster)  [unwired: 9 in]
      n238 = call "Module Name--constant.vi"("Module ID"=w516) -> ("Module Name"=w521:string)  [unwired: 10 in]
      n239 = Format Into String(format string="An error occurred during initialization. %s is no longer running.", w521) -> (resulting string=w519:string)  [unwired: 2 in, 1 out]
      n240 = call "Error Reported.vi"("Additional Information"=w519, "Error"=w523, "Module ID"=w516) -> ()  [unwired: 8 in, 1 out]
    }
  }
  n241 = Merge Errors(w17, w16) -> (w18:errorcluster)
  n242 = call "Close Module.vi"("error in"=w18, "Wait for stop?"=w2, "Module Admin in"=w4) -> ("error out"=w14:errorcluster, "External Launch"=w1:bool, "Module Admin out"=w3:refnum<class "Delacor_lib_QMH_Cloneable Module Admin.lvclass">)  [unwired: 6 in]
  n243 = Unregister For Events(event registration refnum=w9, error in=w14) -> (error out=w13:errorcluster)
  "error out" <- w13
  n244 = case "External Launch?" shown="True" w1 {
    tunnel: w13 -> [_ w525]
    frame False {
    }
    frame True {
      n245 = case shown="No Error" w525 {
        frame No Error {
          n246 = invoke class="VI" method="FP.Close"() -> ()  [unwired: 3 in, 3 out]
        }
        frame Error {
          n247 = disable-structure shown="Default" {
            frame condition #0 (active) {
              n248 = invoke class="VI" method="FP.Open"("Activate"=TRUE ("Activate?")) -> ()  [unwired: 4 in, 5 out]
            }
            frame condition #1 {
              # "Don't show panel on error if running inside a built EXE."
            }
          }
        }
      }
    }
  }
  n249 = local write "Module Admin"(w3) -> ()
